vi "foorloop3.vi"() -> ()   [LabVIEW 2020]
panel:
  out "Elapsed Time (s)":dbl
  in  "Time Target (s)":dbl=40.0
  in  "tiempo de espera":u32
  out "numero aleatorio":dbl
  out "repeticiones":i32
  in  "Numeric":i32
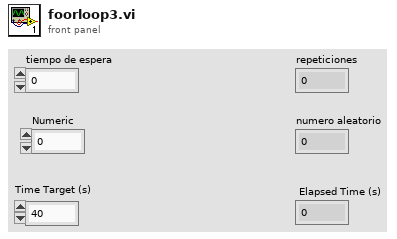
[diagram p1: front panel]
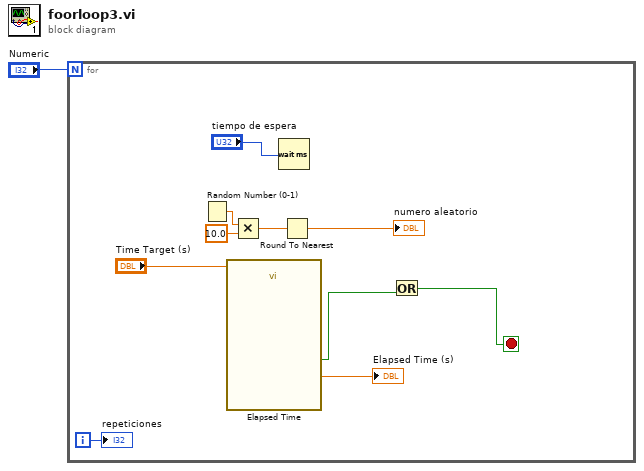
[diagram p0: block diagram]
diagram:
  n1 = for {
    N: "Numeric" -> [_]
    i -> [w11]
    stop <- w5 stop-if-true
    n2 = Random Number (0-1)() -> (number: 0 to 1=w10:dbl)
    n3 = call "Elapsed Time"("Time Target (s)"="Time Target (s)") -> ("Elapsed Time (s)"=→"Elapsed Time (s)":dbl, "Time has Elapsed"=w6:bool)  [unwired: 11 in, 6 out]
    n4 = Multiply(x=w10, y=10.0) -> (x*y=w8:dbl)
    n5 = Wait (ms)(milliseconds to wait="tiempo de espera") -> ()  [unwired: 1 out]
    n6 = Round To Nearest(number=w8) -> (nearest integer value=→"numero aleatorio":dbl)
    n7 = Or(y=w6) -> (x .or. y?=w5:bool)  [unwired: 1 in]
    "repeticiones" <- w11
  }
